vi "Handle Error.vi"(8 "error in (no error)":errorcluster, 11 "Stage Controller in":refnum<class "Stage Controller.lvclass">) -> (0 "error out":errorcluster, 2 "stop actor?":bool=TRUE, 3 "Stage Controller out":refnum<class "Stage Controller.lvclass">)   [LabVIEW 2018, in "Stage Controller.lvlib" / "Stage Controller.lvclass"]
doc: "(<B>Filename</B>: Actor Framework.lvlib:Actor.lvclass:Handle Error.vi)\n\nDefines how the actor handles an error that occurred while processing a message.\n\nBy default, this method does nothing except stop the actor. This method also treats error code 43 (coming from <B>error in</B>) as a sign that the actor shut down normally. In this situation, the Handle Error method does not return the error on <B>error out</B>, meaning the actor's caller will not receive it. All other error codes will be returned on <B>error out</B>.\n\nA descendant class may override this method to change this behavior."
uses:
  Stage Controller.lvclass
  Device/Device.lvclass
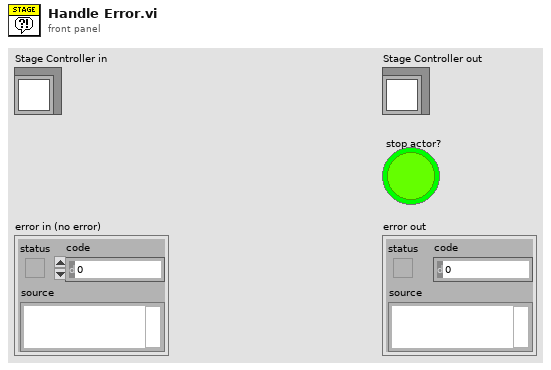
[diagram p1: front panel]
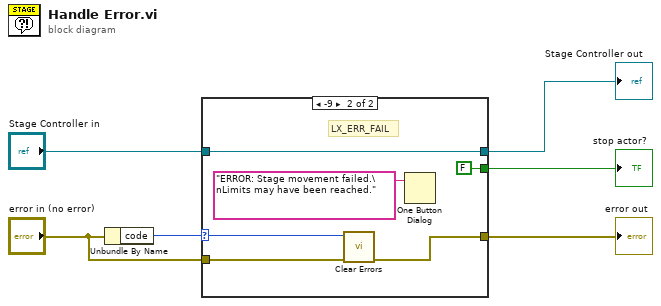
[diagram p0: block diagram]
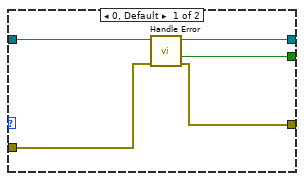
[diagram p2: hidden frame]
diagram:
  n1 = Unbundle By Name("error in (no error)") -> ("code"=w6:i32)
  n2 = case shown="-9" w6 {
    selector: w6 -> [_ w13]
    tunnel: "error in (no error)" -> [w7 w17]
    tunnel: "Stage Controller in" -> [w11 w16]
    tunnel: [w10 w16] -> w3
    tunnel: [w9 FALSE ("stop actor?")] -> w2
    tunnel: [w8 w15] -> w1
    frame 0, Default {
      n3 = call-parent "Handle Error.vi"("error in (no error)"=w7, "Device in"=w11) -> ("error out"=w8:errorcluster, "stop actor?"=w9:bool, "Device out"=w10:refnum<class "Stage Controller.lvclass">)  [unwired: 7 in]
    }
    frame -9 {
      # "LX_ERR_FAIL"
      n4 = call <vilib>:"Clear Errors.vi"("error in (no error)"=w17, "specific error code to clear (0: all)"=w13) -> ("error out"=w15:errorcluster)  [unwired: 4 in, 1 out]
      n5 = One Button Dialog(message="ERROR: Stage movement failed.\nLimits may have been reached.") -> ()  [unwired: 1 in, 1 out]
    }
  }
  "Stage Controller out" <- w3
  "error out" <- w1
  "stop actor?" <- w2
